vi "parse_equations_embedded_in_string.vi"(9 "all variable values (min or calculated)":dbl[](array[numeric]), 10 "all variable names":string[](array[string]), 11 "input $equation$ string":string caption="(if box is checked, may use equations as $x+a0$)") -> (3 "parsed $equation$ string":string)   [LabVIEW 2013]
uses:
  <vilib>/regexp/Match Regular Expression.xnode
  <vilib>/gmath/NI_Gmath.lvlib
panel:
  in  "error in":errorcluster
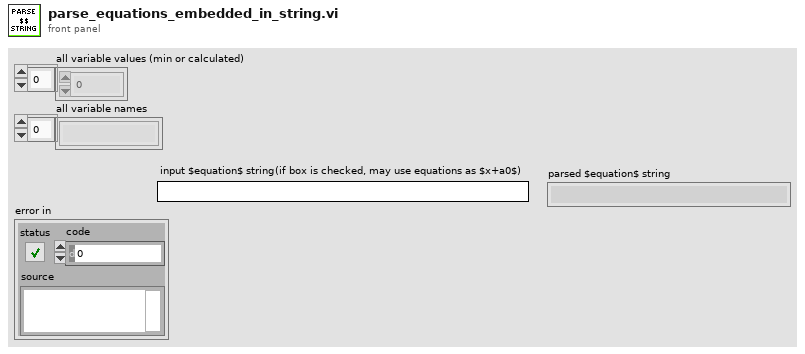
[diagram p1: front panel]
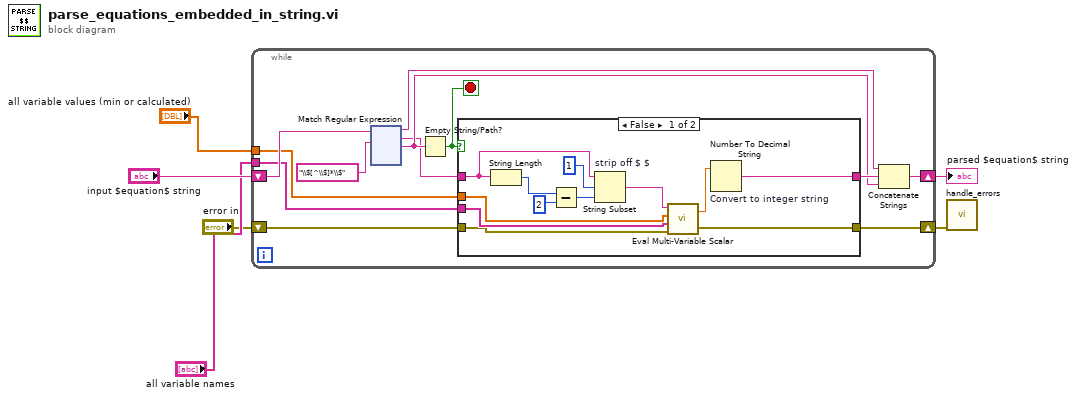
[diagram p0: block diagram]
diagram:
  n1 = while {
    tunnel: "all variable values (min or calculated)" -> [w16]
    tunnel: "all variable names" -> [w15]
    shift-right: [w11] -> w5
    shift-left: "input $equation$ string" -> [w18]
    shift-right: [w7] -> w4
    shift-left: "error in" -> [w8]
    stop <- w9 stop-if-true
    n2 = xnode "Match Regular Expression"("input string"=w18, "regular expression"="\\$[^\\$]*\\$") -> ("before match"=w14:string, "whole match"=w10:string, "after match"=w12:string)  [unwired: 4 in, 2 out]
    n3 = Empty String/Path?(string/path=w12) -> (empty?=w9:bool)
    n4 = case shown="False" w9 {
      tunnel: w10 -> [w29 w32]
      tunnel: w16 -> [w25 _]
      tunnel: w15 -> [w23 _]
      tunnel: [w21 w32] -> w13
      tunnel: w8 -> [w20 w31]
      tunnel: [w19 w31] -> w7
      frame False {
        n5 = String Length(string=w29) -> (length=w28:i32)
        n6 = Subtract(x=w28, y=2) -> (x-y=w27:i32)
        n7 = String Subset "strip off $ $"(string=w29, offset (0)=1, length (rest)=w27) -> (substring=w24:string)
        n8 = call <vilib>:"Eval Multi-Variable Scalar.vi"("error in (no error)"=w20, "Variables"=w23, "X Values"=w25, "formula"=w24) -> ("error out"=w19:errorcluster, "y value"=w22:dbl)
        n9 = Number To Decimal String "Convert to integer string"(number=w22) -> (decimal integer string=w21:string)  [unwired: 1 in]
      }
      frame True {
      }
    }
    n10 = Concatenate Strings(w14, w13, w12) -> (w11:string)
  }
  "parsed $equation$ string" <- w5
  n11 = call "handle_errors.vi"("error in (no error)"=w4) -> ()  [unwired: 10 in, 1 out]
